vi "Swerve_Drive.vi"(0 "Z":dbl(knob) scale=1.0..-1.0, 5 "Y":dbl(slide) scale=1.0..-1.0, 7 "X":dbl(slide)=0.5 scale=-1.0..1.0) -> (2 "Back Left Spin Speed":dbl=-0.0, 3 "Back Right Spin Speed":dbl=-0.0, 4 "Front Left Spin Speed":dbl=-0.0, 6 "Front Right Spin Speed":dbl=-0.0, 8 "Back Left Motor Power":dbl=-0.59, 10 "Back Right Motor Power":dbl=0.5, 14 "Front Right Motor Power":dbl=-0.5, 15 "Front Left Motor Power":dbl=0.59)   [LabVIEW 2018]
uses:
  Global_Variables/Kinematic_Globals.vi
  Global_Variables/Sensor_Values.vi
panel:
  out "FR":T1(graph)
  out "BR":T1(graph)
  out "BL":T1(graph)
  out "FL":T1(graph)
  in  "Back_Right":bool=TRUE
  in  "Front_Right":bool=TRUE
  in  "Front_Left":bool=TRUE
  in  "Back_Left":bool=TRUE
  in  "Kp":dbl=0.01495
  # "0.01425"
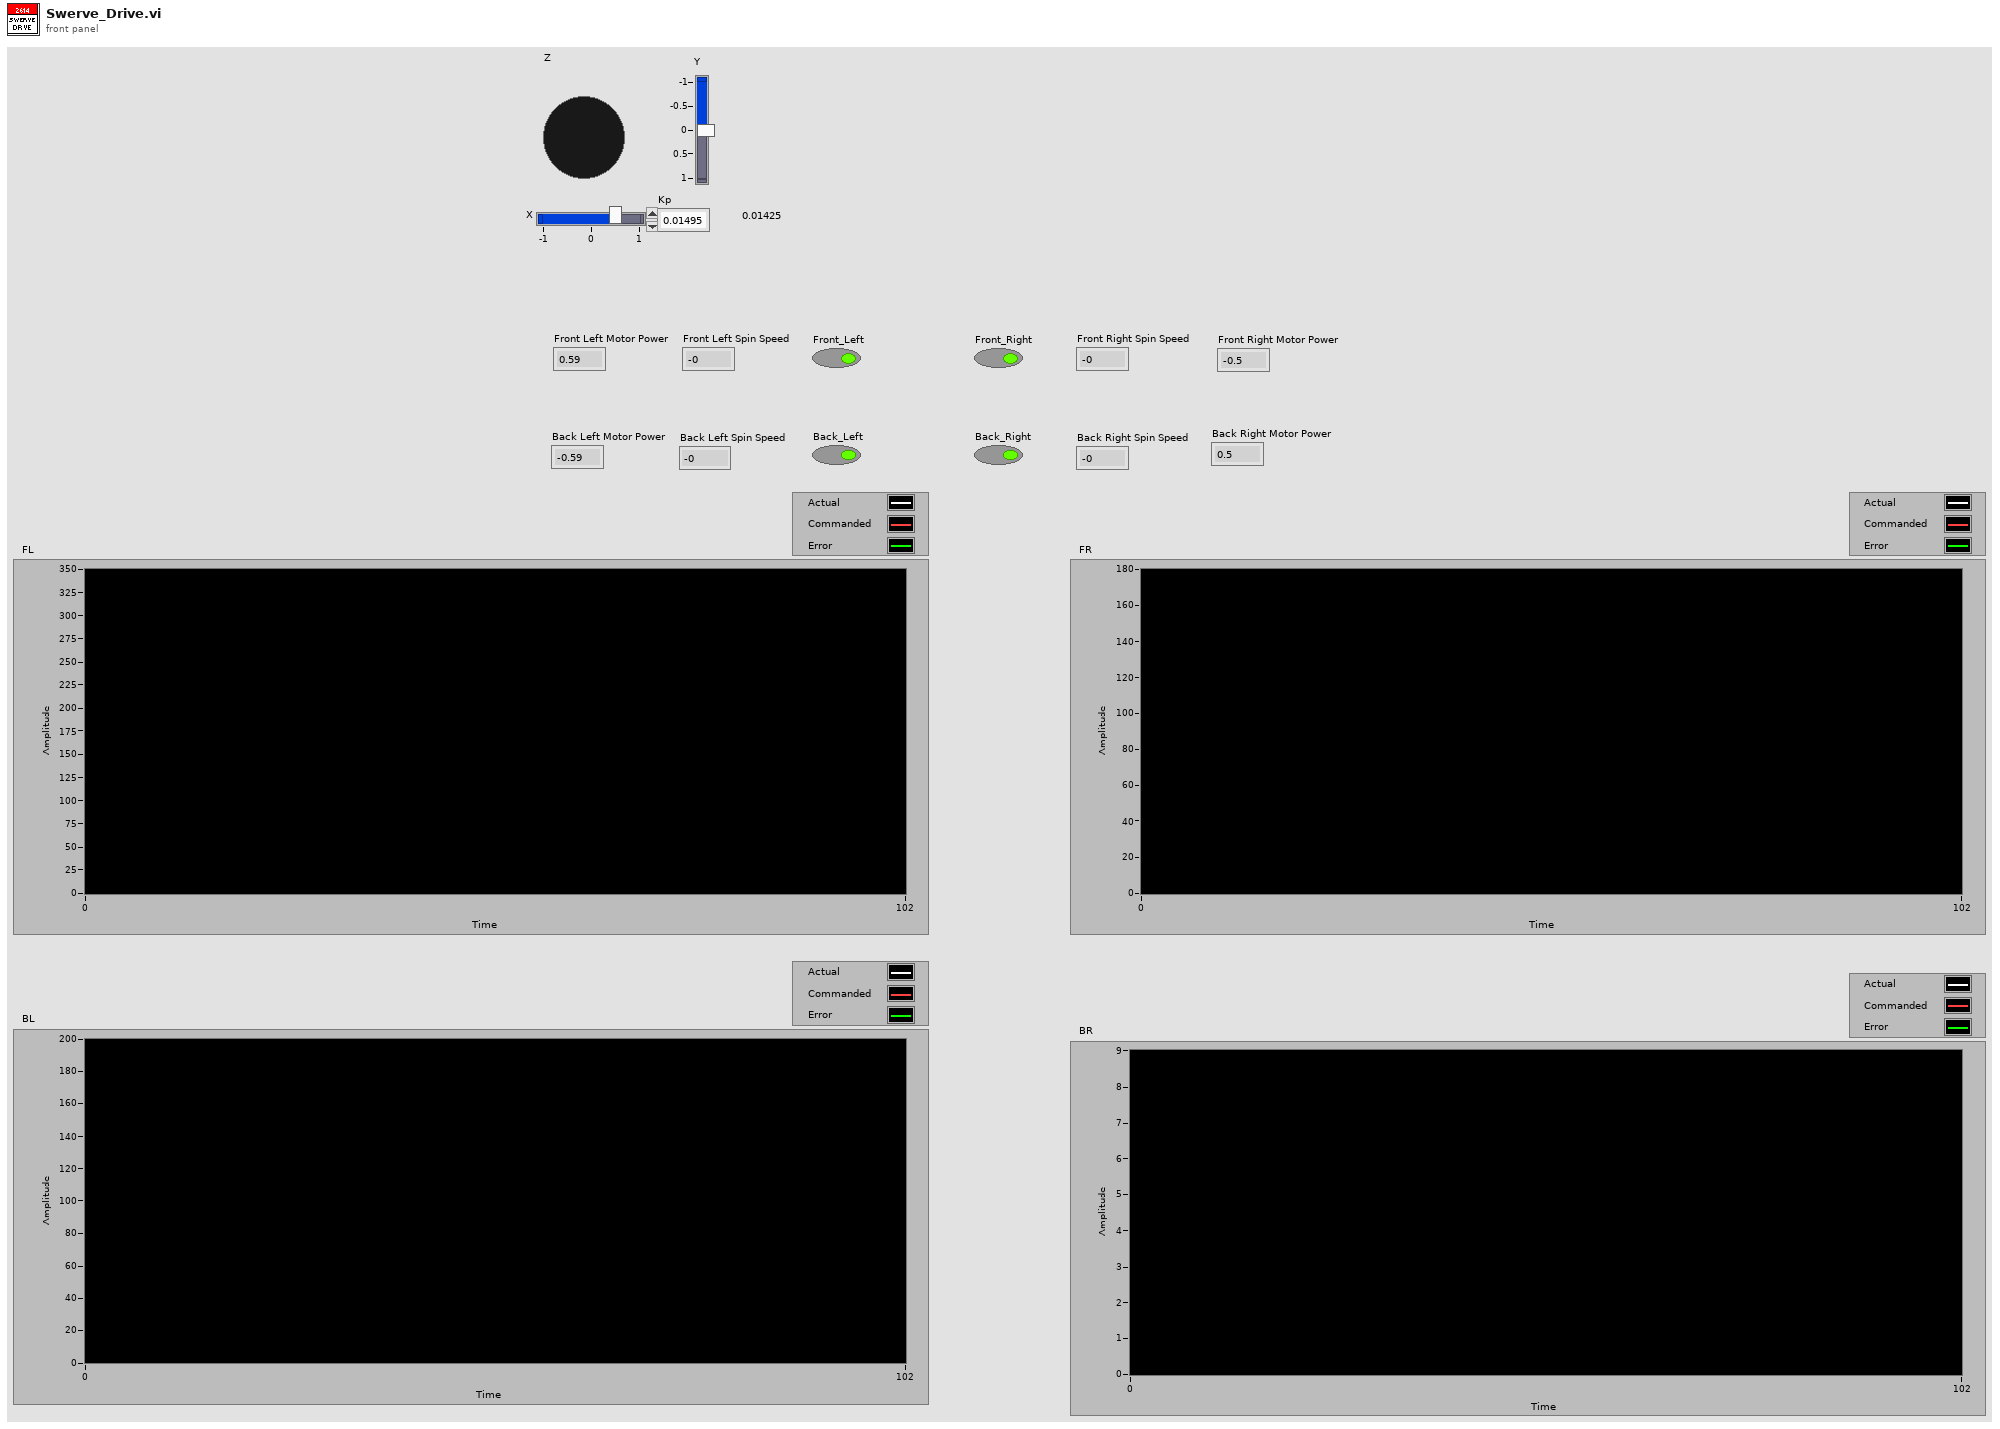
[diagram p1: front panel]
types:
  T1 = cluster{"Front Left Wheel Angle":dbl, dbl, "Error":dbl}
  T2 = cluster{"Back_Right_Azimuth":dbl, "Angle_Goal":dbl, dbl}
  T3 = cluster{"Front_Right_Azimuth":dbl, "Angle_Goal":dbl, dbl}
  T4 = cluster{"Back_Left_Azimuth":dbl, "Angle_Goal":dbl, dbl}
  T5 = cluster{"Front_Left_Azimuth":dbl, "Angle_Goal":dbl, dbl}
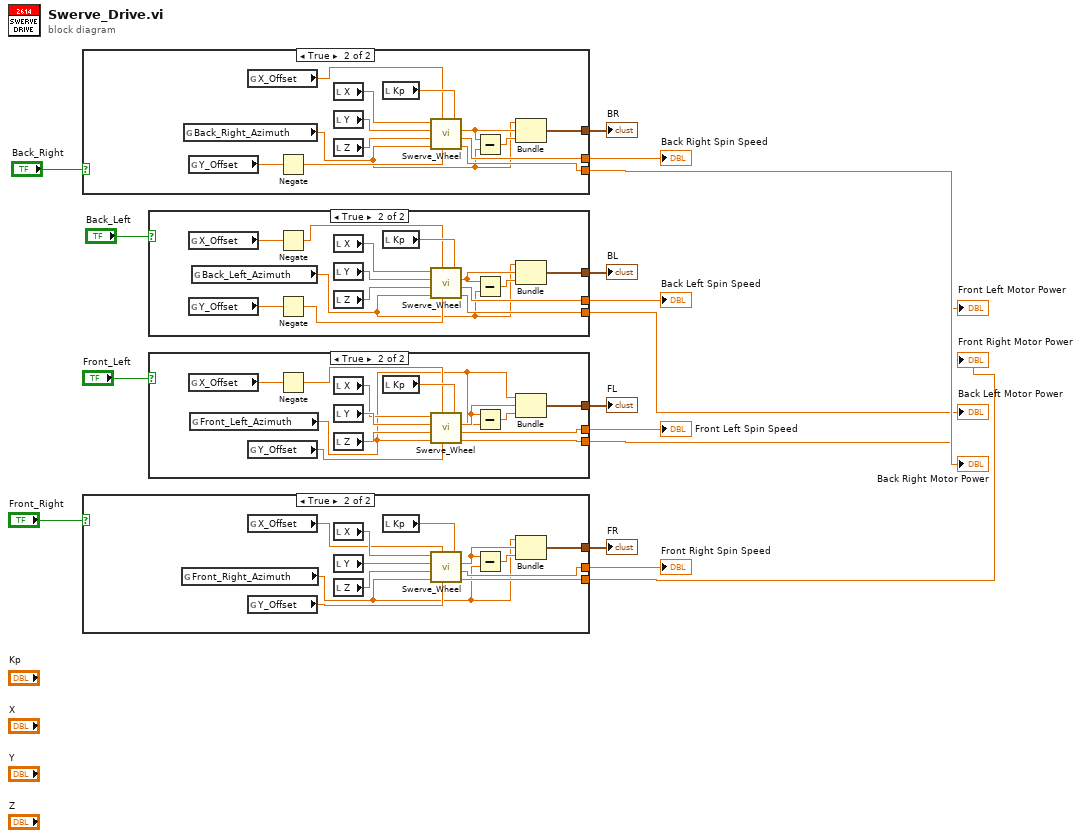
[diagram p0: block diagram]
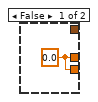
[diagram p2: hidden frame]
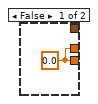
[diagram p3: hidden frame]
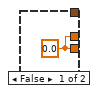
[diagram p4: hidden frame]
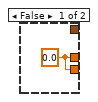
[diagram p5: hidden frame]
diagram:
  n1 = case shown="True" "Back_Right" {
    tunnel: [w17 w30] -> w10
    tunnel: [w17 w29] -> w4
    tunnel: [_ w24] -> w7
    frame False {
      w17 = 0.0
    }
    frame True {
      n2 = global read "Sensor_Values.vi" "Back_Right_Azimuth"() -> (w18:dbl)
      n3 = global read "Kinematic_Globals.vi" "Y_Offset"() -> (w21:dbl)
      n4 = global read "Kinematic_Globals.vi" "X_Offset"() -> (w19:dbl)
      n5 = Negate(x=w21) -> (-x=w20:dbl)
      n6 = local read "X"() -> (w27:dbl)
      n7 = local read "Y"() -> (w26:dbl)
      n8 = local read "Z"() -> (w25:dbl)
      n9 = local read "Kp"() -> (w28:dbl)
      n10 = call "Swerve_Wheel.vi"("Kp"=w28, "Offset_Y"=w20, "Offset_X"=w19, "Wheel_Angle"=w18, "Z"=w25, "Y"=w26, "X"=w27) -> ("Wheel_Speed"=w29:dbl, "Turn_Speed"=w30:dbl, "Angle_Goal"=w22:dbl)
      n11 = Subtract(x=w22, y=w18) -> (x-y=w23:dbl)
      n12 = Bundle("Back_Right_Azimuth"=w18, "Angle_Goal"=w22, w23) -> (w24:T2)  [unwired: 1 in]
    }
  }
  "Back Right Spin Speed" <- w10
  "Back Right Motor Power" <- w4
  "BR" <- w7
  n13 = case shown="True" "Front_Right" {
    tunnel: [w31 w43] -> w11
    tunnel: [w31 w42] -> w1
    tunnel: [_ w37] -> w8
    frame False {
      w31 = 0.0
    }
    frame True {
      n14 = global read "Sensor_Values.vi" "Front_Right_Azimuth"() -> (w32:dbl)
      n15 = global read "Kinematic_Globals.vi" "X_Offset"() -> (w33:dbl)
      n16 = global read "Kinematic_Globals.vi" "Y_Offset"() -> (w34:dbl)
      n17 = local read "X"() -> (w38:dbl)
      n18 = local read "Y"() -> (w39:dbl)
      n19 = local read "Z"() -> (w40:dbl)
      n20 = local read "Kp"() -> (w41:dbl)
      n21 = call "Swerve_Wheel.vi"("Kp"=w41, "Offset_Y"=w34, "Offset_X"=w33, "Wheel_Angle"=w32, "Z"=w40, "Y"=w39, "X"=w38) -> ("Wheel_Speed"=w42:dbl, "Turn_Speed"=w43:dbl, "Angle_Goal"=w35:dbl)
      n22 = Subtract(x=w35, y=w32) -> (x-y=w36:dbl)
      n23 = Bundle("Front_Right_Azimuth"=w32, "Angle_Goal"=w35, w36) -> (w37:T3)  [unwired: 1 in]
    }
  }
  "Front Right Motor Power" <- w1
  "Front Right Spin Speed" <- w11
  "FR" <- w8
  n24 = case shown="True" "Back_Left" {
    tunnel: [w44 w58] -> w12
    tunnel: [w44 w57] -> w3
    tunnel: [_ w52] -> w6
    frame False {
      w44 = 0.0
    }
    frame True {
      n25 = global read "Kinematic_Globals.vi" "X_Offset"() -> (w47:dbl)
      n26 = global read "Kinematic_Globals.vi" "Y_Offset"() -> (w49:dbl)
      n27 = global read "Sensor_Values.vi" "Back_Left_Azimuth"() -> (w45:dbl)
      n28 = Negate(x=w47) -> (-x=w46:dbl)
      n29 = Negate(x=w49) -> (-x=w48:dbl)
      n30 = local read "X"() -> (w53:dbl)
      n31 = local read "Y"() -> (w54:dbl)
      n32 = local read "Z"() -> (w55:dbl)
      n33 = local read "Kp"() -> (w56:dbl)
      n34 = call "Swerve_Wheel.vi"("Kp"=w56, "Offset_Y"=w48, "Offset_X"=w46, "Wheel_Angle"=w45, "Z"=w55, "Y"=w54, "X"=w53) -> ("Wheel_Speed"=w57:dbl, "Turn_Speed"=w58:dbl, "Angle_Goal"=w50:dbl)
      n35 = Subtract(x=w50, y=w45) -> (x-y=w51:dbl)
      n36 = Bundle("Back_Left_Azimuth"=w45, "Angle_Goal"=w50, w51) -> (w52:T4)  [unwired: 1 in]
    }
  }
  "Back Left Motor Power" <- w3
  "Back Left Spin Speed" <- w12
  "BL" <- w6
  n37 = case shown="True" "Front_Left" {
    tunnel: [w59 w72] -> w2
    tunnel: [w59 w71] -> w9
    tunnel: [_ w66] -> w5
    frame False {
      w59 = 0.0
    }
    frame True {
      n38 = global read "Kinematic_Globals.vi" "X_Offset"() -> (w62:dbl)
      n39 = global read "Sensor_Values.vi" "Front_Left_Azimuth"() -> (w60:dbl)
      n40 = global read "Kinematic_Globals.vi" "Y_Offset"() -> (w63:dbl)
      n41 = Negate(x=w62) -> (-x=w61:dbl)
      n42 = local read "X"() -> (w67:dbl)
      n43 = local read "Y"() -> (w68:dbl)
      n44 = local read "Z"() -> (w69:dbl)
      n45 = local read "Kp"() -> (w70:dbl)
      n46 = call "Swerve_Wheel.vi"("Kp"=w70, "Offset_Y"=w63, "Offset_X"=w61, "Wheel_Angle"=w60, "Z"=w69, "Y"=w68, "X"=w67) -> ("Wheel_Speed"=w72:dbl, "Turn_Speed"=w71:dbl, "Angle_Goal"=w64:dbl)
      n47 = Subtract(x=w64, y=w60) -> (x-y=w65:dbl)
      n48 = Bundle("Front_Left_Azimuth"=w60, "Angle_Goal"=w64, w65) -> (w66:T5)  [unwired: 1 in]
    }
  }
  "Front Left Motor Power" <- w2
  "Front Left Spin Speed" <- w9
  "FL" <- w5
